vi "ReadTestItems(SubVI).vi"(8 "error in (no error)":errorcluster, 10 "Model path":path, 11 "VI in":refnum<vi>) -> (0 "error out":errorcluster, 2 "items out":string[][](array[string]), 3 "VI out":refnum<vi>)   [LabVIEW 2013]
uses:
  <vilib>/regexp/Match Regular Expression.xnode
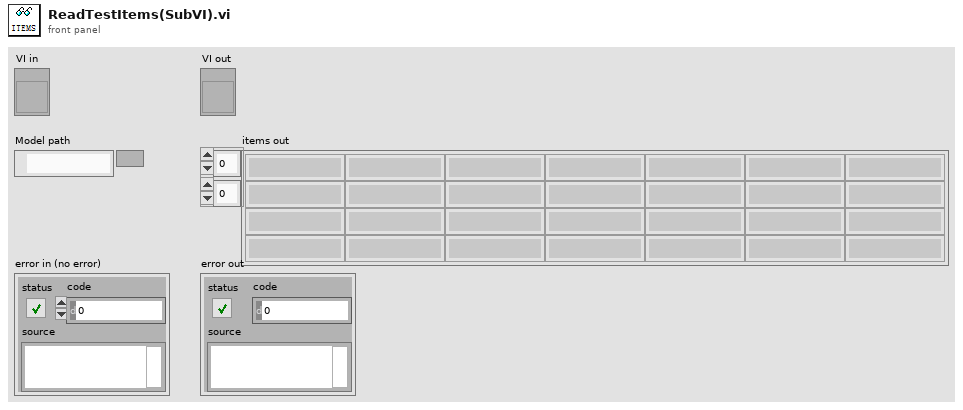
[diagram p1: front panel]
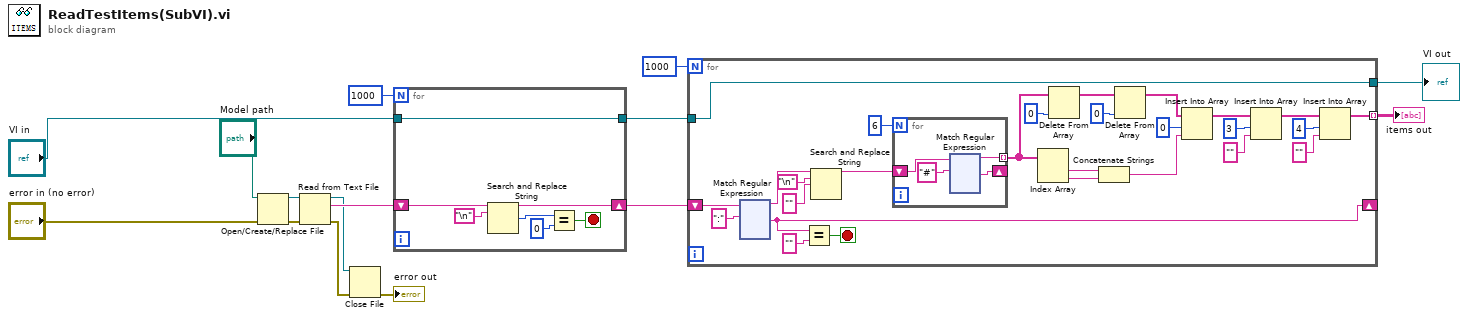
[diagram p0: block diagram]
diagram:
  n1 = Open/Create/Replace File(file path (use dialog)="Model path", error in="error in (no error)") -> (refnum out=w2:refnum<file>, error out=w1:errorcluster)  [unwired: 4 in, 1 out]
  n2 = Read from Text File(file (use dialog)=w2, error in=w1) -> (refnum out=w5:refnum<file>, text=w7:string, error out=w4:errorcluster)  [unwired: 2 in, 1 out]
  n3 = Close File(refnum=w5, error in=w4) -> (error out=→"error out":errorcluster)  [unwired: 1 out]
  n4 = for {
    N: 1000 -> [_]
    shift-right: [w20] -> w8
    shift-left: w7 -> [w21]
    tunnel: "VI in" -> [w16]
    tunnel: [w16] -> w13
    stop <- w17 stop-if-true
    n5 = Search and Replace String(input string=w21, search string="\n") -> (result string=w20:string, number of replacements=w19:i32)  [unwired: 6 in, 2 out]
    n6 = Equal?(x=w19, y=0) -> (x = y?=w17:bool)
  }
  n7 = for {
    N: 1000 -> [_]
    shift-right: [w30] -> _
    shift-left: w8 -> [w49]
    tunnel: [w31] -> w9 mode=indexing
    tunnel: w13 -> [w23]
    tunnel: [w23] -> w14
    stop <- w28 stop-if-true
    n8 = xnode ("Match Regular Expression")("input string"=w49, "regular expression"=":") -> ("before match"=w27:string, "after match"=w30:string)  [unwired: 4 in, 3 out]
    n9 = Equal?(x=w30, y="") -> (x = y?=w28:bool)
    n10 = Search and Replace String(input string=w27, search string="\n" ("Line Feed Constant"), replace string="" ("replace string (\"\")")) -> (result string=w24:string)  [unwired: 5 in, 3 out]
    n11 = for {
      N: 6 -> [_]
      shift-right: [w51] -> _
      shift-left: w24 -> [w52]
      tunnel: [w50] -> w44 mode=indexing
      n12 = xnode "Match Regular Expression"("input string"=w52, "regular expression"="#") -> ("before match"=w50:string, "after match"=w51:string)  [unwired: 4 in, 3 out]
    }
    n13 = Index Array(array=w44) -> (element #1=w45:string, element #2=w46:string)  [unwired: 2 in]
    n14 = Delete From Array(array=w44, index=0) -> (array with subset deleted=w43:string[])  [unwired: 1 in, 1 out]
    n15 = Concatenate Strings(w45, w46) -> (w39:string)
    n16 = Delete From Array(array=w43, index=0) -> (array with subset deleted=w40:string[])  [unwired: 1 in, 1 out]
    n17 = Insert Into Array(array=w40, index=0, new element=w39) -> (w37:string[])
    n18 = Insert Into Array(array=w37, index=3, new element="" ("new element/subarray")) -> (w34:string[])
    n19 = Insert Into Array(array=w34, index=4, new element="" ("new element/subarray")) -> (w31:string[])
  }
  "items out" <- w9
  "VI out" <- w14
